vi "Roborealm Connect Set Camera.vi"(4 "remote port or service name":u16=1180, 6 "UP IP Address":string, 7 "Camera":string, 8 "error in (no error)":errorcluster, 9 "Width":string, 10 "Height":string) -> (0 "error out":errorcluster, 2 "connection ID out":refnum<k5>)   [LabVIEW 2017]
panel:
  out "output 2":string
  out "offset past scan":u32
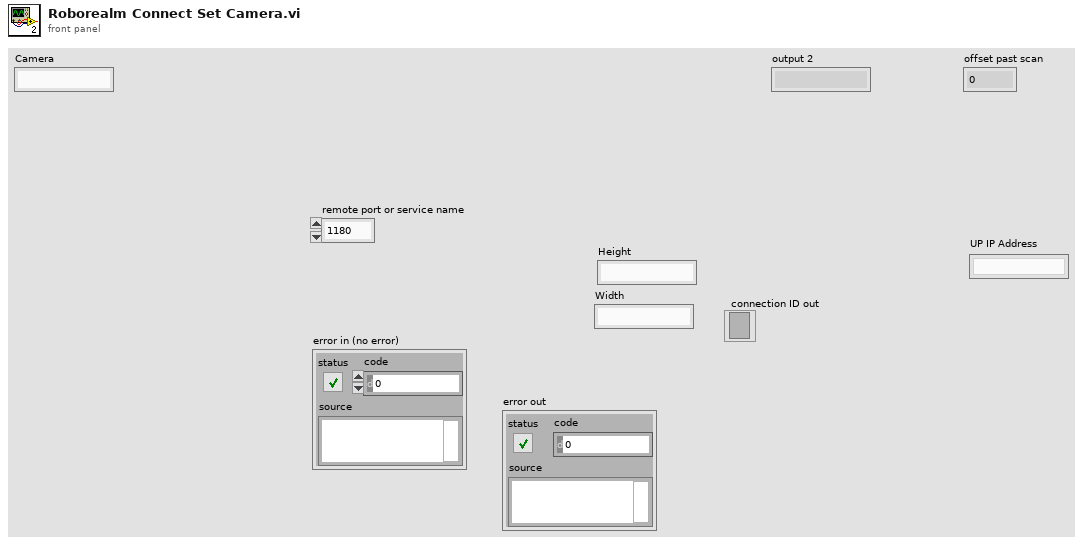
[diagram p1: front panel]
types:
  T1 = enum16{"Standard", "Buffered", "CRLF", "Immediate"}
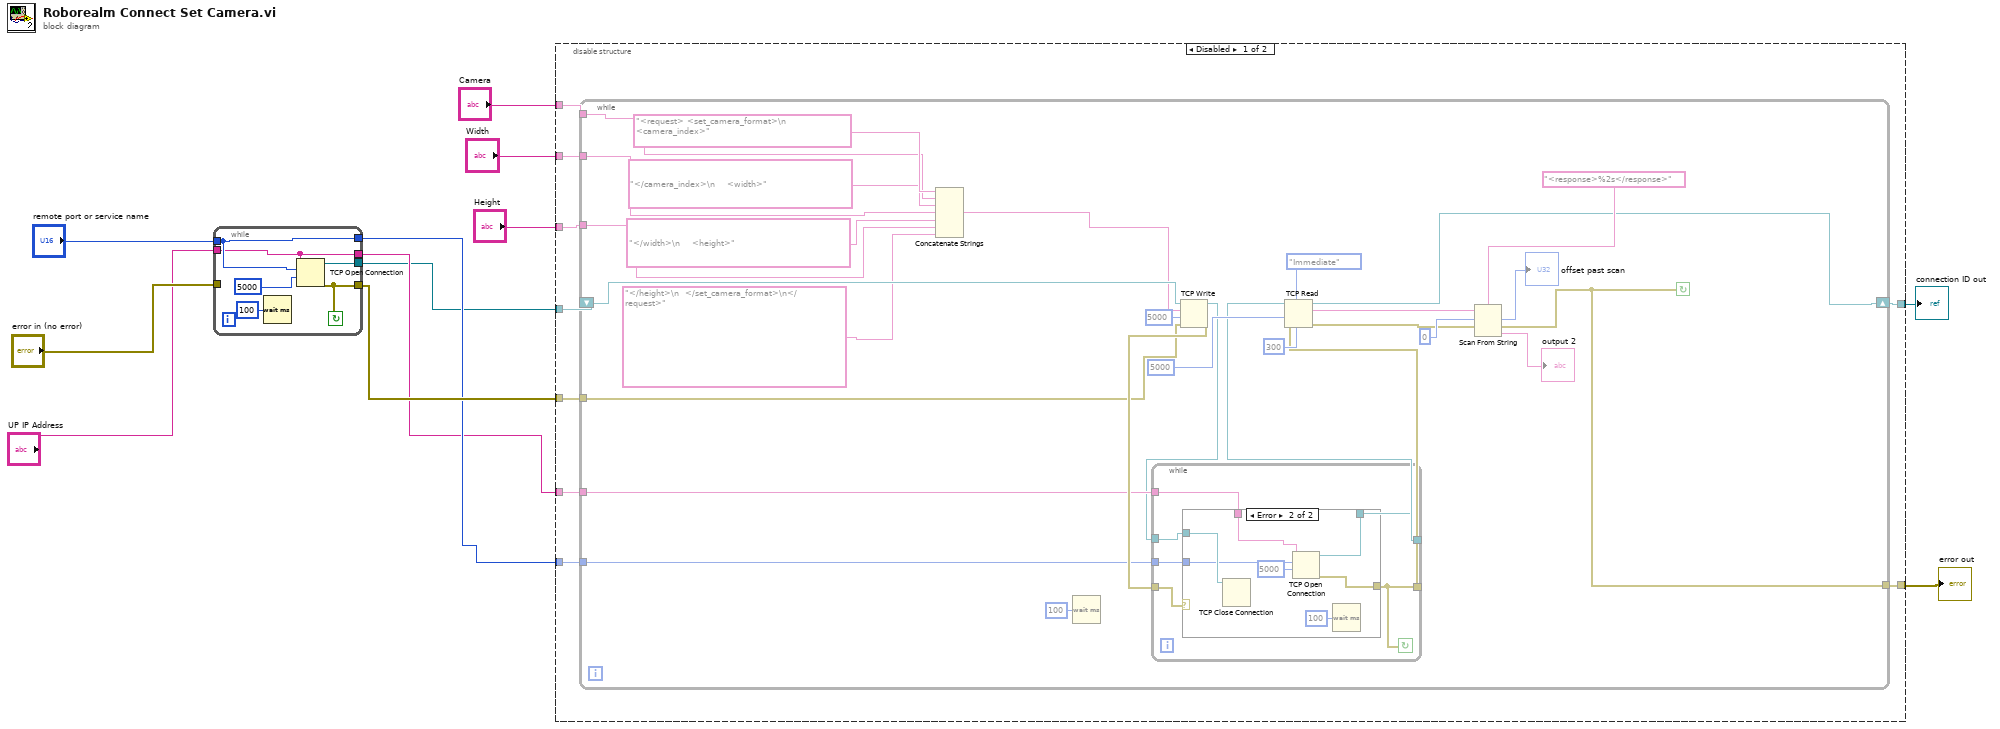
[diagram p0: block diagram]
diagram:
  n1 = while {
    tunnel: "error in (no error)" -> [_]
    tunnel: [w17] -> w7
    tunnel: [w13] -> w3
    tunnel: [w14] -> w6
    tunnel: [w16] -> w2
    tunnel: "remote port or service name" -> [w14]
    tunnel: "UP IP Address" -> [w13]
    stop <- w17 continue-if-true
    n2 = Wait (ms)(milliseconds to wait=u32 100) -> ()  [unwired: 1 out]
    n3 = TCP Open Connection(address=w13, remote port or service name=w14, timeout ms (60000)=5000) -> (connection ID=w16:refnum<k5>, error out=w17:errorcluster)  [unwired: 2 in]
  }
  n4 = disable-structure shown="Disabled" {
    disable-tunnel: [w27 w73] -> w12
    disable-tunnel: "Width" -> [w26 _]
    disable-tunnel: "Height" -> [w25 _]
    disable-tunnel: "Camera" -> [w24 _]
    disable-tunnel: w7 -> [w23 w72]
    disable-tunnel: w6 -> [w22 _]
    disable-tunnel: w3 -> [w21 _]
    disable-tunnel: w2 -> [w20 w73]
    disable-tunnel: [w19 w72] -> w1
    frame Disabled {
      n5 = while {
        shift-right: [w37] -> w27
        shift-left: w20 -> [w47]
        tunnel: w21 -> [w45]
        tunnel: w23 -> [w46]
        tunnel: [w38] -> w19
        tunnel: w22 -> [w40]
        tunnel: w26 -> [w32]
        tunnel: w25 -> [w31]
        tunnel: w24 -> [w34]
        stop <- w38 continue-if-true
        n6 = Concatenate Strings("<request> <set_camera_format>\n    <camera_index>" ("data in"), w34, "</camera_index>\n    <width>" ("data in"), w32, "</width>\n    <height>" ("data in"), w31, "</height>\n  </set_camera_format>\n</request>" ("data in")) -> (w28:string)
        n7 = Wait (ms)(milliseconds to wait=u32 100) -> ()  [unwired: 1 out]
        n8 = TCP Write(connection ID=w47, data in=w28, error in (no error)=w46, 9:5000 ("timeout ms (25000)")) -> (connection ID out=w43:refnum<k5>, error out=w49:errorcluster)  [unwired: 1 out]
        n9 = while {
          tunnel: w45 -> [w60]
          tunnel: [w59] -> w42
          tunnel: w43 -> [w58]
          tunnel: w49 -> [w62]
          tunnel: [w61] -> w48
          tunnel: w40 -> [w57]
          stop <- w61 continue-if-true
          n10 = case shown="Error" w62 {
            selector: w62 -> [w64 _]
            tunnel: [w64 w70] -> w61
            tunnel: [w63 w69] -> w59
            tunnel: w58 -> [w63 w67]
            tunnel: w60 -> [_ w68]
            tunnel: w57 -> [_ w66]
            frame No Error {
            }
            frame Error {
              n11 = TCP Close Connection(connection ID=w67) -> ()  [unwired: 2 in, 2 out]
              n12 = TCP Open Connection(address=w68, remote port or service name=w66, timeout ms (60000)=5000) -> (connection ID=w69:refnum<k5>, error out=w70:errorcluster)  [unwired: 2 in]
              n13 = Wait (ms)(milliseconds to wait=u32 100) -> ()  [unwired: 1 out]
            }
          }
        }
        n14 = TCP Read(connection ID=w42, bytes to read=300, error in (no error)=w48, 7:T1."Immediate" ("mode (standard)"), 9:5000 ("bytes to read")) -> (connection ID out=w37:refnum<k5>, data out=w50:string, error out=w51:errorcluster)
        n15 = Scan From String(format string="<response>%2s</response>", input string=w50, initial scan location=u32 0, error in=w51) -> (offset past scan=→"offset past scan":u32, error out=w38:errorcluster, output 1=→"output 2":string)  [unwired: 1 in, 1 out]
      }
    }
    frame Enabled {
    }
  }
  "error out" <- w1
  "connection ID out" <- w12
